vi "Create_Default_Destinations.vi"(8 "error in (no error)":errorcluster, 9 "Destination Name":string, 10 "Destination Path":path, 11 "AB_Application in":refnum<class "AB_Application.lvclass">) -> (0 "error out":errorcluster, 2 "default dests":refnum<class "AB_Destination.lvclass">[](array[class]), 3 "AB_Application out":refnum<class "AB_Application.lvclass">)   [LabVIEW 2020, in "AB_Application.lvclass"]
uses:
  <vilib>/AppBuilder/AB_Classes/Application/AB_Application.lvclass
  <vilib>/AppBuilder/AB_Classes/Destination/AB_Destination.lvclass
  <resource>/Framework/Providers/Common/provcom_StringGlobals.vi
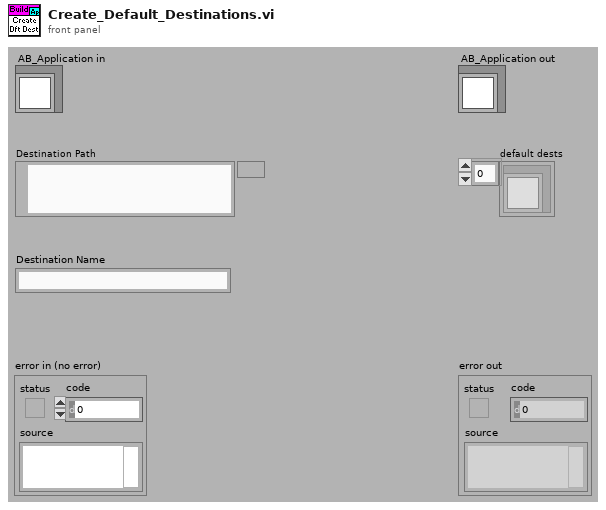
[diagram p1: front panel]
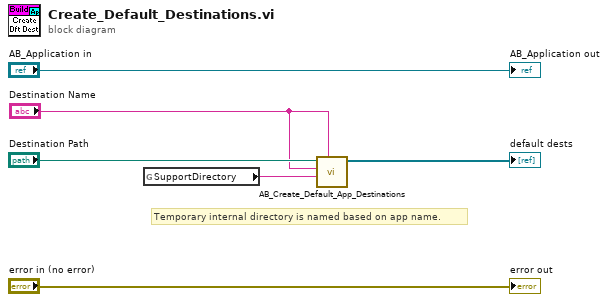
[diagram p0: block diagram]
diagram:
  # "Temporary internal directory is named based on app name."
  n1 = global read "provcom_StringGlobals.vi" "SupportDirectory"() -> (w6:string)
  n2 = call <vilib>:"AB_Create_Default_App_Destinations.vi"("internal dir name"="Destination Name", "SupportDirectory"=w6, "App Name"="Destination Name", "App Destination Path"="Destination Path") -> ("default app dests"=→"default dests":refnum<class "AB_Destination.lvclass">[])  [unwired: 2 in, 5 out]
  "error out" <- "error in (no error)"
  "AB_Application out" <- "AB_Application in"
